vi "niDTS BT INSTR TX Configure Trigger.vi"(8 "error in (no error)":errorcluster, 11 "niDTS BT INSTR TX in":refnum<class "niDTS BT INSTR TX.lvclass">) -> (0 "error out":errorcluster, 3 "niDTS BT INSTR TX out":refnum<class "niDTS BT INSTR TX.lvclass">)   [LabVIEW 2015, in "niDTS BT.lvlib" / "niDTS BT INSTR TX.lvclass"]
doc: "Sets:\n\n* TriggerThreshold\n* Trigger Source\n* MinQuietTimeDuration\n* TriggerTimeout"
uses:
  niDTS BT INSTR TX.lvclass
  niDTS BT INSTR TX.lvclass/niDTS BT INSTR TX.ctl
  RiviInstDriver/niRfsaBT/Objects/niRfsaBt.lvclass
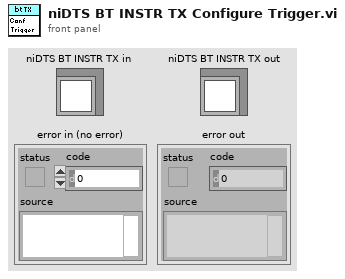
[diagram p1: front panel]
types:
  T1 = typedef "niRfsaBT.lvclass/niRfsaBT INC Handle.ctl" = refnum<data-value>
  T2 = enum16{"IMMediate", "RF0", "PFI0", "PFI1", "RTS0", "RTS1", "RTS2", "RTS3", "RTS4", "RTS5", "RTS6", "RTS7", "PXIStar", "SOFT"}
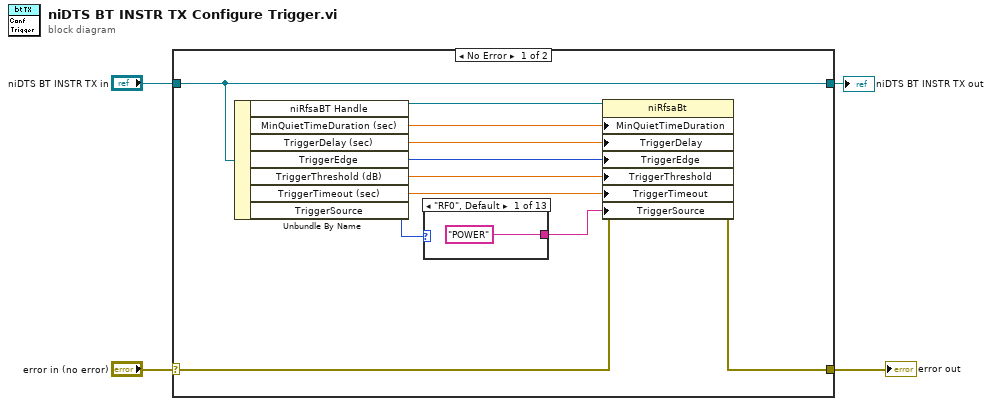
[diagram p0: block diagram]
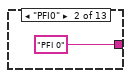
[diagram p2: hidden frame]
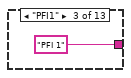
[diagram p3: hidden frame]
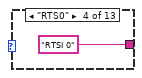
[diagram p4: hidden frame]
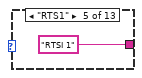
[diagram p5: hidden frame]
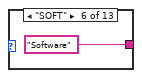
[diagram p6: hidden frame]
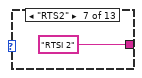
[diagram p7: hidden frame]
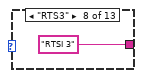
[diagram p8: hidden frame]
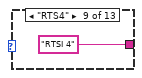
[diagram p9: hidden frame]
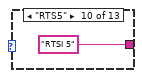
[diagram p10: hidden frame]
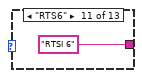
[diagram p11: hidden frame]
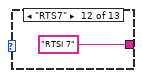
[diagram p12: hidden frame]
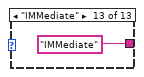
[diagram p13: hidden frame]
diagram:
  n1 = case shown="No Error" "error in (no error)" {
    selector: "error in (no error)" -> [w15 w30]
    tunnel: [w14 w30] -> w3
    tunnel: "niDTS BT INSTR TX in" -> [w5 w29]
    tunnel: [w5 w29] -> w1
    frame No Error {
      n2 = Unbundle By Name(w5) -> ("niRfsaBT Handle"=w13:T1, "MinQuietTimeDuration (sec)"=w8:dbl, "TriggerDelay (sec)"=w9:dbl, "TriggerEdge"=w10:enum16{"RISing", "FALLing"}, "TriggerThreshold (dB)"=w11:dbl, "TriggerTimeout (sec)"=w12:dbl, "TriggerSource"=w7:T2)
      n3 = case shown="\"RF0\", Default" w7 {
        tunnel: ["POWER" ("TRIGger:RFSA:BLUetooth:TriggerSource") "PFI 0" ("TRIGger:RFSA:BLUetooth:TriggerSource") "PFI 1" ("TRIGger:RFSA:BLUetooth:TriggerSource") "RTSI 0" ("TRIGger:RFSA:BLUetooth:TriggerSource") "RTSI 1" ("TRIGger:RFSA:BLUetooth:TriggerSource") "Software" ("TRIGger:RFSA:BLUetooth:TriggerSource") "RTSI 2" ("TRIGger:RFSA:BLUetooth:TriggerSource") "RTSI 3" ("TRIGger:RFSA:BLUetooth:TriggerSource") "RTSI 4" ("TRIGger:RFSA:BLUetooth:TriggerSource") "RTSI 5" ("TRIGger:RFSA:BLUetooth:TriggerSource") "RTSI 6" ("TRIGger:RFSA:BLUetooth:TriggerSource") "RTSI 7" ("TRIGger:RFSA:BLUetooth:TriggerSource") "IMMediate" ("TRIGger:RFSA:BLUetooth:TriggerSource")] -> w6
        frame "RF0", Default {
        }
        frame "PFI0" {
        }
        frame "PFI1" {
        }
        frame "RTS0" {
        }
        frame "RTS1" {
        }
        frame "SOFT" {
        }
        frame "RTS2" {
        }
        frame "RTS3" {
        }
        frame "RTS4" {
        }
        frame "RTS5" {
        }
        frame "RTS6" {
        }
        frame "RTS7" {
        }
        frame "IMMediate" {
        }
      }
      n4 = property class="niRfsaBt"(reference=w13, error in=w15, "MinQuietTimeDuration"=w8, "TriggerDelay"=w9, "TriggerEdge"=w10, "TriggerThreshold"=w11, "TriggerTimeout"=w12, "TriggerSource"=w6) -> (error out=w14:errorcluster)  [unwired: 1 out]
    }
    frame Error {
    }
  }
  "error out" <- w3
  "niDTS BT INSTR TX out" <- w1
